vi "AOM_XY.vi"(11 "In":waveform(dbl)) -> (3 "Out":waveform(dbl))   [LabVIEW 2018]
uses:
  <vilib>/measure/NI_MABase.lvlib
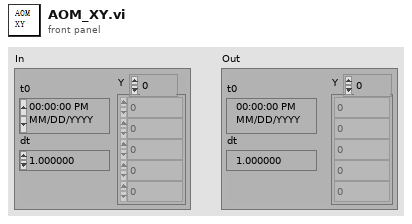
[diagram p1: front panel]
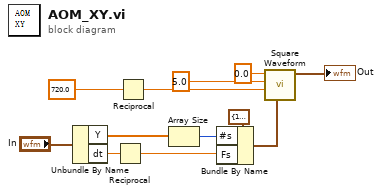
[diagram p0: block diagram]
diagram:
  n1 = Unbundle By Name("In") -> ("Y"=w5:dbl[], "dt"=w9:dbl)
  n2 = Reciprocal(x=w9) -> (1/x=w10:dbl)
  n3 = Reciprocal(x=720.0 ("phase")) -> (1/x=w1:dbl)
  n4 = Array Size(array=w5) -> (size(s)=w8:i32)
  n5 = Bundle By Name(cluster=cluster{"Fs":dbl, "#s":dbl} {"Fs"=1000.0, "#s"=1000.0} ("sampling info"), "#s"=w8, "Fs"=w10) -> (w7:cluster{"Fs":dbl, "#s":dbl})
  n6 = call <vilib>:"Square Waveform.vi"("sampling info"=w7, "phase"=w1, "amplitude"=5.0, "frequency"=0.0) -> ("signal out"=→"Out":waveform(dbl))  [unwired: 6 in, 1 out]
